vi "Delete Bucket Policy.vi"(8 "error in (no error)":errorcluster, 11 "Bucket in":refnum<class "Bucket.lvclass">) -> (0 "error out":errorcluster, 3 "Bucket out":refnum<class "Bucket.lvclass">)   [LabVIEW 2015, in "NI_AWS_S3.lvlib" / "Bucket.lvclass"]
doc: "This implementation of the DELETE operation uses the policy subresource to delete the policy on a specified bucket. To use the operation, you must have DeletePolicy permissions on the specified bucket and be the bucket owner.\n\nIf you do not have DeletePolicy permissions, Amazon S3 returns a 403 Access Denied error. If you have the correct permissions, but are not a user of the bucket owner account, Amazon S3 returns a 405 Method Not Allowed error. If the bucket doesn't have a policy, Amazon S3 returns a 204 No Content error. There are restrictions about who can create bucket policies and which objects in a bucket they can apply to."
uses:
  Bucket.lvclass
  Core/HTTP Request/Region handling.ctl
  Core/HTTP Request/Request Options.ctl
  Core/HTTP Request/Name Value Pair.ctl
  Core/HTTP Request/URL formatting.ctl
  Bucket.lvclass/Bucket.ctl
  Read Name.vi
  Core/HTTP Request/HTTP Request.lvclass
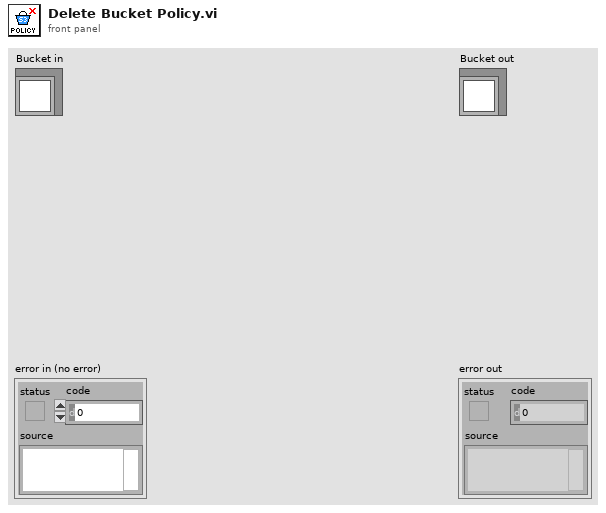
[diagram p1: front panel]
types:
  T1 = typedef "NI_AWS_Core.lvlib/HTTP Request.lvclass/Name Value Pair.ctl" = cluster{"name":string, "value":string}
  T2 = typedef "NI_AWS_Core.lvlib/HTTP Request.lvclass/Request Options.ctl" = cluster{"request headers":T1[], "request parameters":T1[], "request body":string, "region handling":T3, "URL formatting":T4}
  T3 = typedef "NI_AWS_Core.lvlib/HTTP Request.lvclass/Region handling.ctl" = enum16{"use region everywhere", "use region (authentication only)", "use region (URL only)", "ignore region everwhere"}
  T4 = typedef "NI_AWS_Core.lvlib/HTTP Request.lvclass/URL formatting.ctl" = enum16{"region-", "region."}
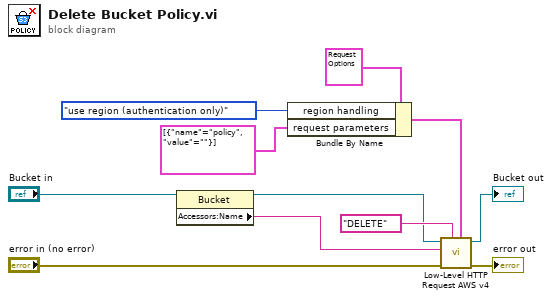
[diagram p0: block diagram]
diagram:
  n1 = property class="Bucket"(reference="Bucket in") -> (reference out=w2:refnum<class "Bucket.lvclass">, "Accessors:Name"=w11:string)  [unwired: 1 in, 1 out]
  n2 = Bundle By Name(cluster=T2 {"request headers"=[], "request parameters"=[], "request body"="", "region handling"=enum."use region everywhere", "URL formatting"=enum."region."} ("Request Options"), "region handling"=Region_handling."use region (authentication only)", "request parameters"=T1[] [{"name"="policy", "value"=""}]) -> (w1:T2)
  n3 = call "Low-Level HTTP Request AWS v4.vi"("Request Options"=w1, "HTTP-Verb"="DELETE", "error in (no error)"="error in (no error)", "URL Prefix"=w11, "AWS Core in"=w2) -> ("error out"=→"error out":errorcluster, "AWS Core out"=→"Bucket out":refnum<class "Bucket.lvclass">)  [unwired: 3 in, 2 out]
